vi "Build_Dashboard.vi"(9 "All Driver Commands":T1, 10 "All_Outputs":T4, 11 "All_Sensor_Readings":T7) -> (3 "PacketToDriverStation":T11)   [LabVIEW 2012]
uses:
  DStoPCPacketTypeDef.ctl
  All_Commands.ctl
  Cirular Shooter/circular_shooter_commands.ctl
  Climber/Climber_Commands.ctl
  All_Outputs.ctl
  Cirular Shooter/Shooter_Outputs.ctl
  Climber/Climber_Outputs.ctl
  All_Sensor_Readings.ctl
  Climber/climber_sensor_readings.ctl
  Cirular Shooter/Shooter_inputs.ctl
  Field Drive/Field_Drive_out.ctl
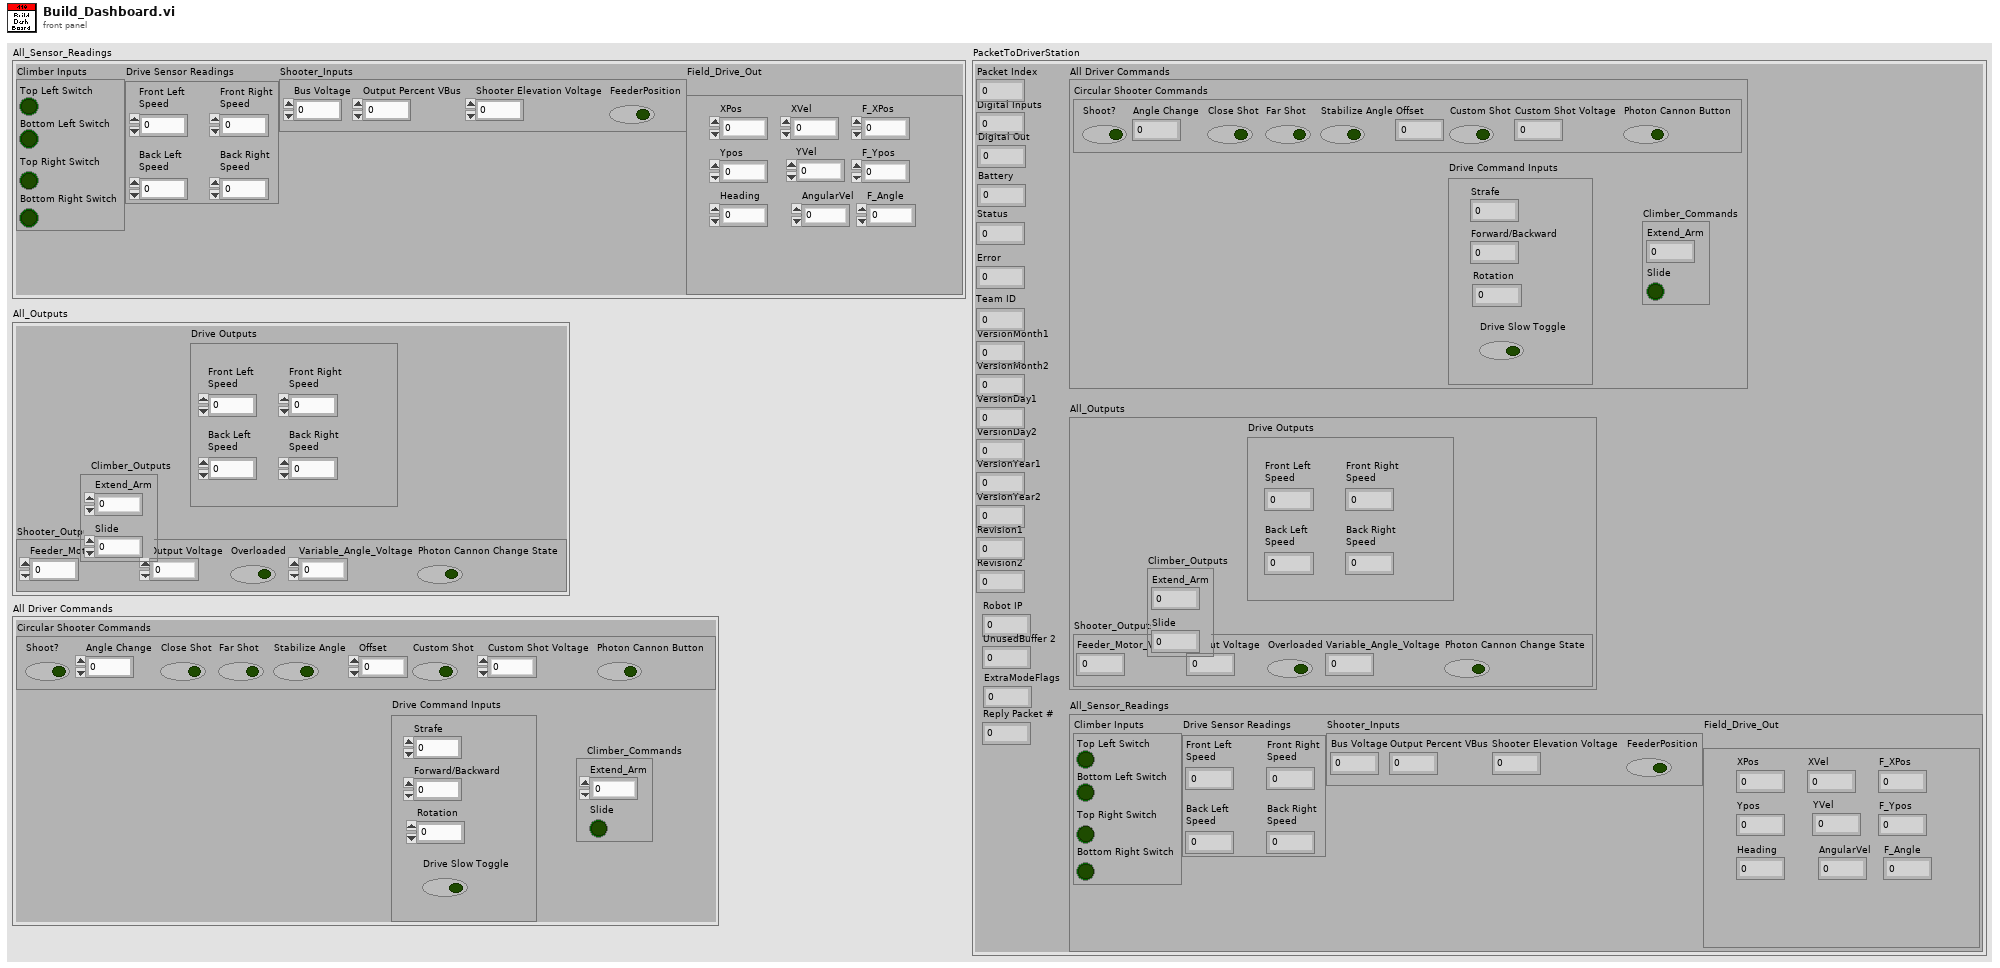
[diagram p1: front panel]
types:
  T1 = typedef "All_Commands.ctl" = cluster{"Circular Shooter Commands":T2, "Drive Command Inputs":cluster{"Strafe":dbl, "Forward/Backward":dbl, "Rotation":dbl, "Drive Slow Toggle":bool}, "Climber_Commands":T3}
  T2 = typedef "circular_shooter_commands.ctl" = cluster{"Shoot?":bool, "Angle Change":dbl, "Close Shot":bool, "Far Shot":bool, "Stabilize Angle ":bool, "Offset":dbl, "Custom Shot":bool, "Custom Shot Voltage":dbl, "Photon Cannon Button":bool}
  T3 = typedef "Climber_Commands.ctl" = cluster{"Extend_Arm":dbl, "Slide":bool}
  T4 = typedef "All_Outputs.ctl" = cluster{"Drive Outputs":cluster{"Front Left\nSpeed":dbl, "Back Left\nSpeed":dbl, "Front Right\nSpeed":dbl, "Back Right\nSpeed":dbl}, "Shooter_Outputs":T5, "Climber_Outputs":T6}
  T5 = typedef "Shooter_Outputs.ctl" = cluster{"Feeder_Motor_Voltage":dbl, "Output Voltage":dbl, "Overloaded":bool, "Variable_Angle_Voltage":dbl, "Photon Cannon Change State":bool}
  T6 = typedef "Climber_Outputs.ctl" = cluster{"Extend_Arm":dbl, "Slide":dbl}
  T7 = typedef "All_Sensor_Readings.ctl" = cluster{"Climber Inputs":T8, "Drive Sensor Readings":cluster{"Front Left\nSpeed":dbl, "Back Left\nSpeed":dbl, "Front Right\nSpeed":dbl, "Back Right\nSpeed":dbl}, "Shooter_Inputs":T9, "Field_Drive_Out\n":T10}
  T8 = typedef "climber_sensor_readings.ctl" = cluster{"Top Left Switch":bool, "Bottom Left Switch":bool, "Top Right Switch":bool, "Bottom Right Switch":bool}
  T9 = typedef "Shooter_inputs.ctl" = cluster{"Bus Voltage":dbl, "Output Percent VBus":dbl, "Shooter Elevation Voltage":dbl, "FeederPosition":bool}
  T10 = typedef "Field_Drive_out.ctl" = cluster{"XPos":dbl, "Ypos":dbl, "XVel":dbl, "YVel":dbl, "Heading":dbl, "AngularVel":dbl, "F_XPos":dbl, "F_Ypos":dbl, "F_Angle":dbl}
  T11 = typedef "DStoPCPacketTypeDef.ctl" = cluster{"Packet Index":u16, "Digital Inputs":u8, "Digital Out":u8, "Battery":u16, "Status":u8, "Error":u8, "Team ID":u16, "VersionMonth1":u8, "VersionMonth2":u8, "VersionDay1":u8, "VersionDay2":u8, "VersionYear1":u8, "VersionYear2":u8, "Revision1":u8, "Revision2":u8, "Robot IP":u32, "UnusedBuffer 2":u8, "ExtraModeFlags":u8, "Reply Packet #":u16, "All Driver Commands":T1, "All_Outputs":T4, "All_Sensor_Readings":T7}
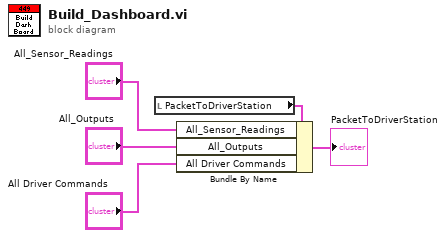
[diagram p0: block diagram]
diagram:
  n1 = local read "PacketToDriverStation"() -> (w4:T11)
  n2 = Bundle By Name(cluster=w4, "All_Sensor_Readings"="All_Sensor_Readings", "All_Outputs"="All_Outputs", "All Driver Commands"="All Driver Commands") -> (→"PacketToDriverStation":T11)
